vi "ConfigYscales.vi"(4 "Language":refnum<vi>, 5 "曲线自定义封存数组":refnum<vi>, 6 "已选数量":refnum<vi>, 7 "Y轴手配":refnum<vi>, 8 "Y标尺总数":i32, 9 "曲线手配":refnum<vi>, 10 "已选信号列表":refnum<vi>) -> ()   [LabVIEW 2015]
uses:
  Ctrls/btnSeeOrNot.ctl
panel:
  out "txtYlink":string
  out "txtUnit":string
  out "txtCurves":string
  out "txtYVisable":string
  out "txtSignal":string
  out "txtRename":string
  out "txtYName":string
  out "txtYsn":string
  out "txtYSetupTitle":string caption="txtYSetup"
  out "txtCurvesSetup":string
  in  "btnSaveCurvesSetup":bool
  in  "曲线配置簇数组":T1(array[cluster]) {"关联Y轴" min=1 max=8 format="Y轴%d"; "曲线序号" format="曲线%d"}
  in  "btnSaveYsetup":bool
  in  "btnExit":bool
  in  "曲线簇":T2={"曲线序号"=0, "SignalName"="", "SignalTag"="", "自定义名"="", "单位"="", "关联Y轴"=1} {"关联Y轴" min=1 max=8 format="Y轴%d"; "曲线序号" format="曲线%d"}
  in  "Y簇":cluster{"Y轴名称 2":string, "Y轴序号 2":i32, "可见性":T3} {"Y轴序号 2" format="Y轴%d"}
  in  "Y轴配置":T4(array[cluster]) {"Y轴序号 2" format="Y轴%d"}
  in  "曲线配置簇":T2
  in  "Y轴配置簇":cluster{"Y轴序号":u8, "Y轴名称":string, "可见性":bool}
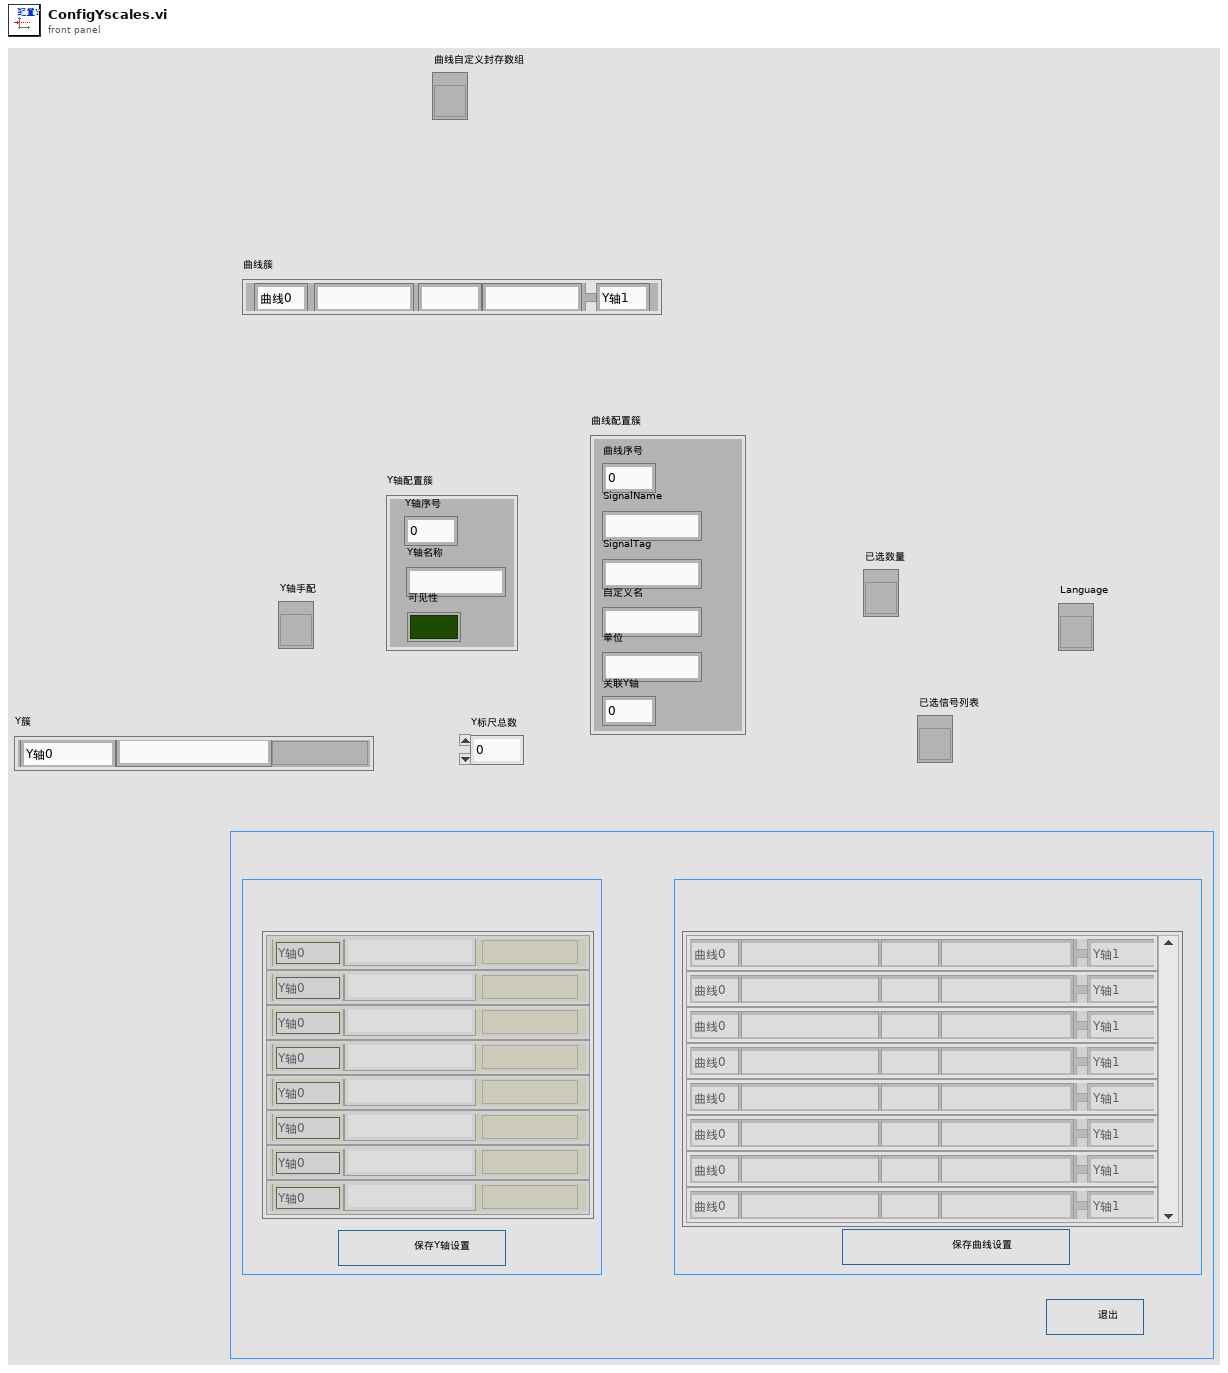
[diagram p1: front panel]
types:
  T1 = cluster{"曲线序号":u8, "SignalName":string, "SignalTag":string, "自定义名":string, "单位":string, "关联Y轴":u8}[]
  T2 = cluster{"曲线序号":u8, "SignalName":string, "SignalTag":string, "自定义名":string, "单位":string, "关联Y轴":u8}
  T3 = typedef "btnSeeOrNot.ctl" = bool
  T4 = cluster{"Y轴名称 2":string, "Y轴序号 2":i32, "可见性":T3}[]
  T5 = enum8{"Enabled", "Disabled", "Disabled and Grayed Out"}
  T6 = typedef "可不可见.ctl" = bool
  T7 = cluster{"Y轴名称 2":string, "Y轴序号 2":i32, "可见性":T6}[]
  T8 = cluster{"曲线序号":u8, "SignalName":string, "SignalTag":string, "自定义名":string, "单位":string, "关联Y轴":u8, "插值方式":dbl}[]
  T9 = cluster{"曲线序号":u8, "SignalName":string, "SignalTag":string, "自定义名":string, "单位":string, "关联Y轴":u8, "插值方式":dbl}
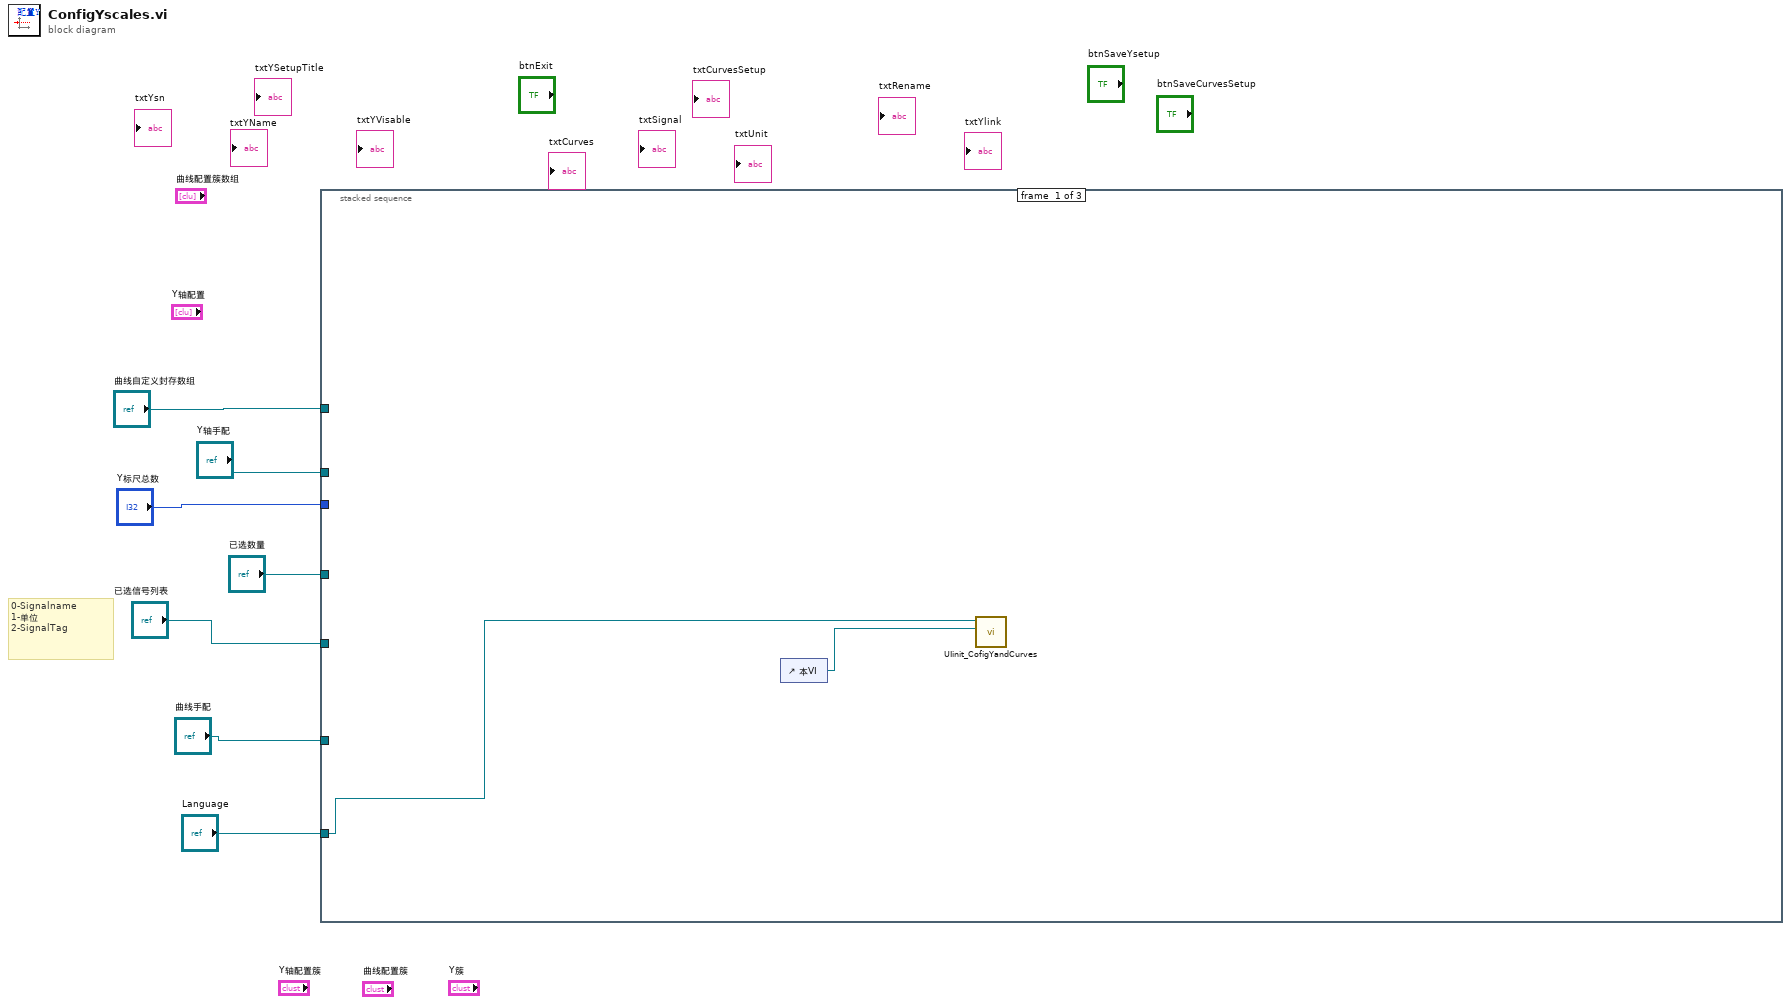
[diagram p0: block diagram]
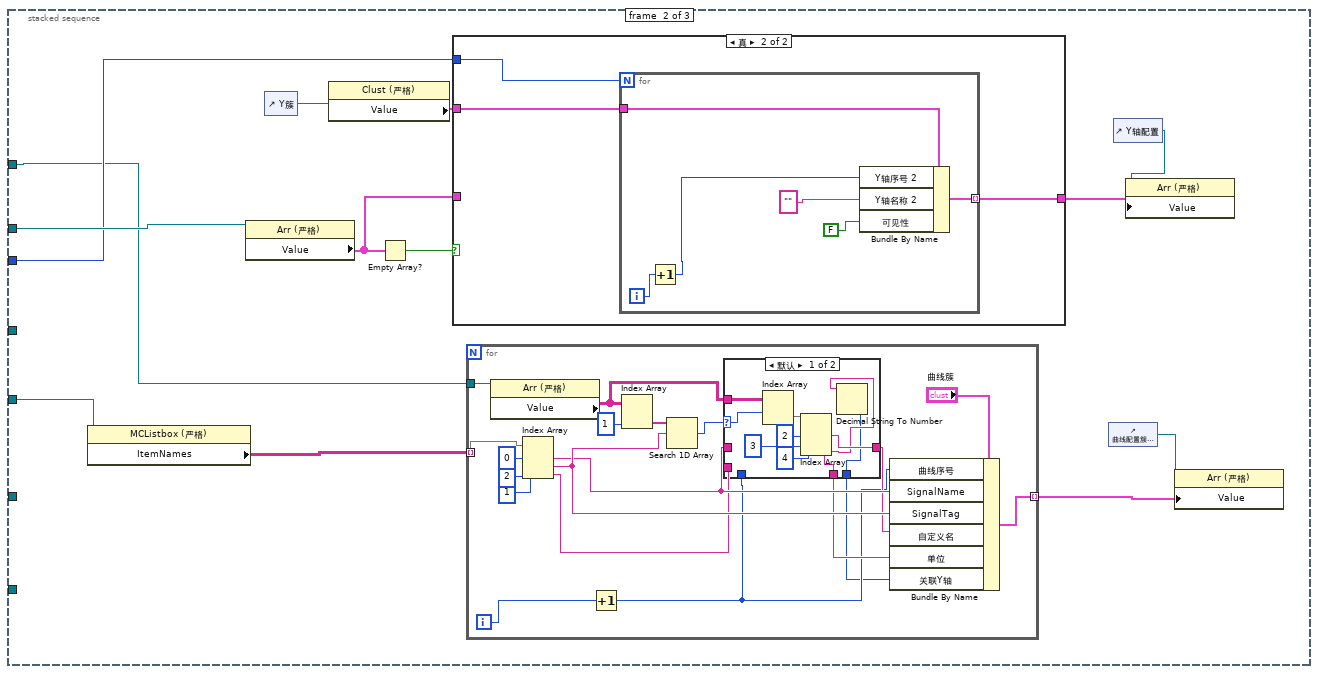
[diagram p2: hidden frame]
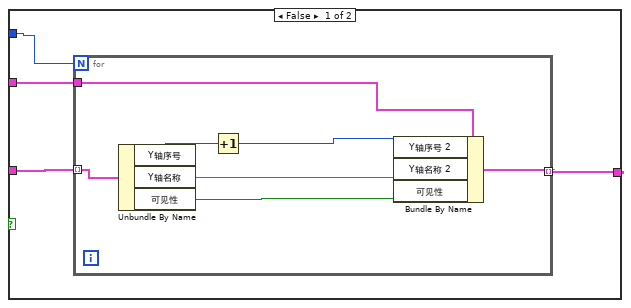
[diagram p4: hidden frame]
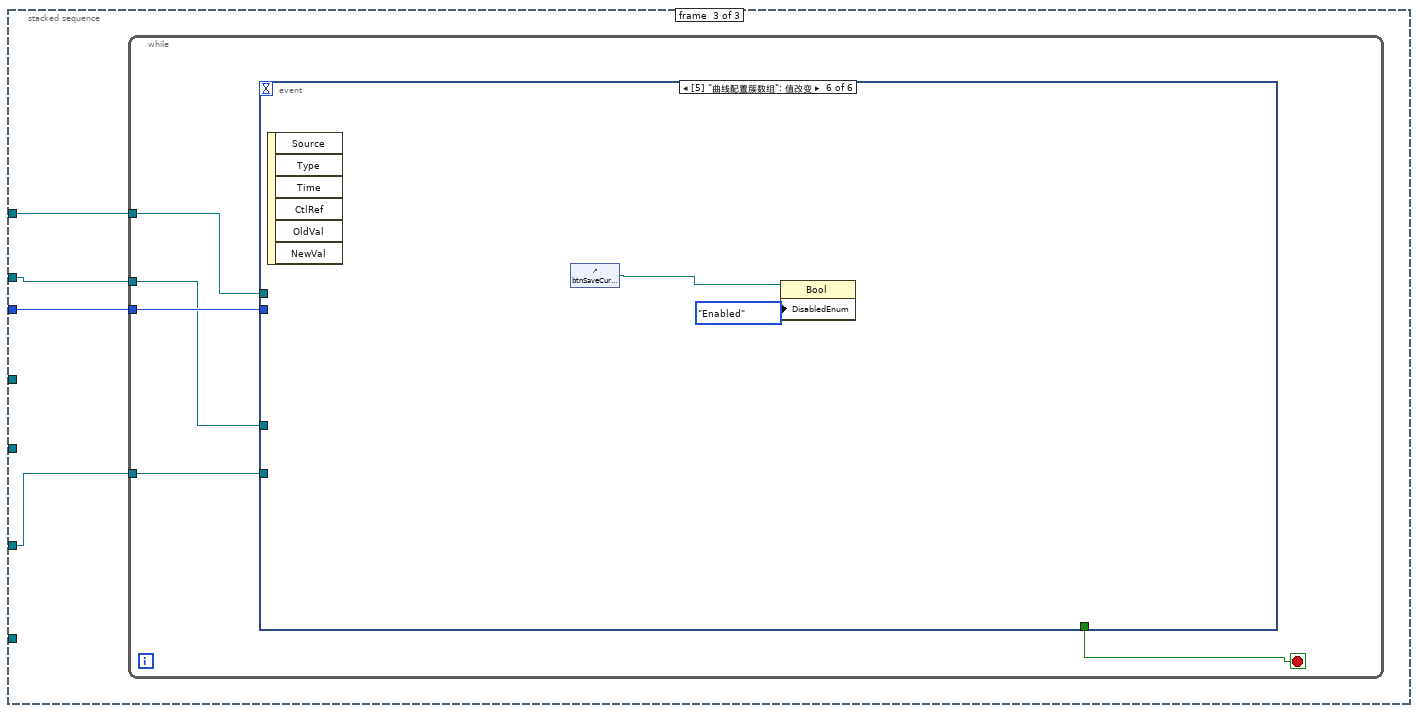
[diagram p5: hidden frame]
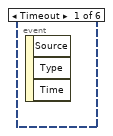
[diagram p6: hidden frame]
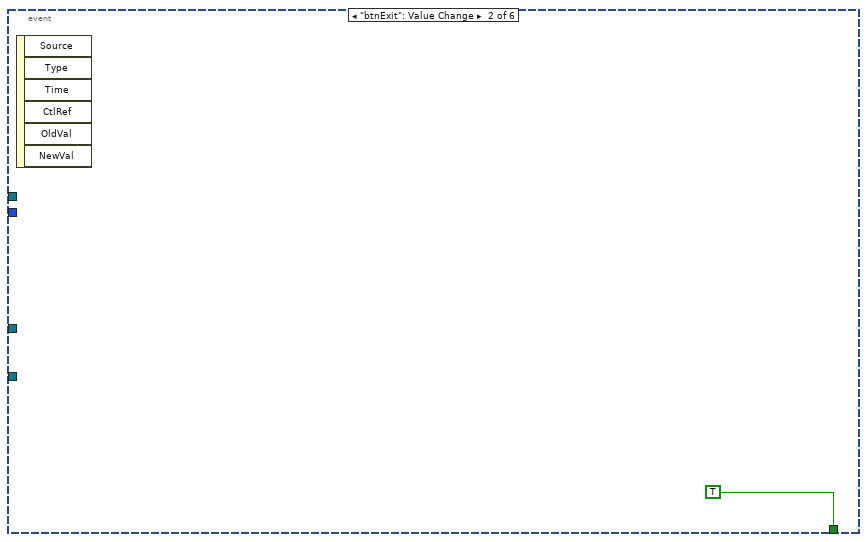
[diagram p7: hidden frame]
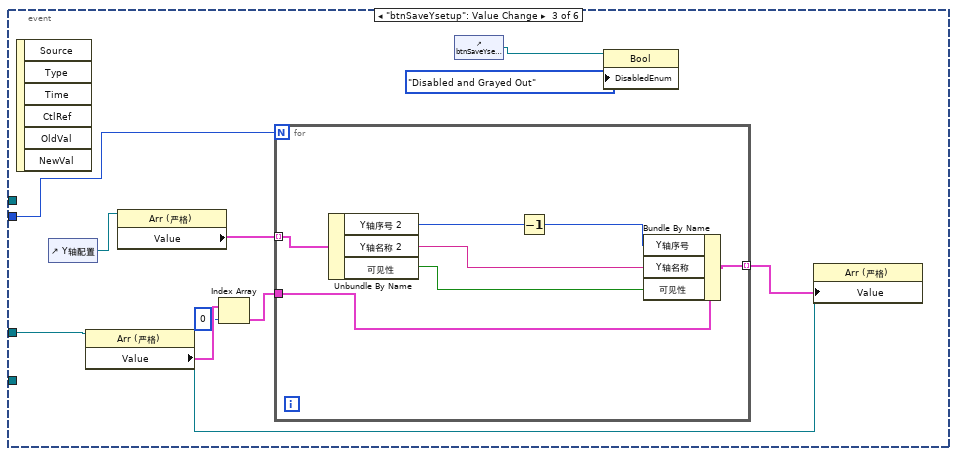
[diagram p8: hidden frame]
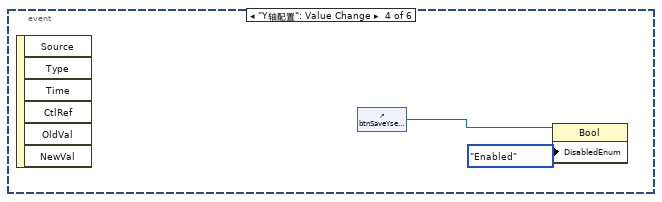
[diagram p9: hidden frame]
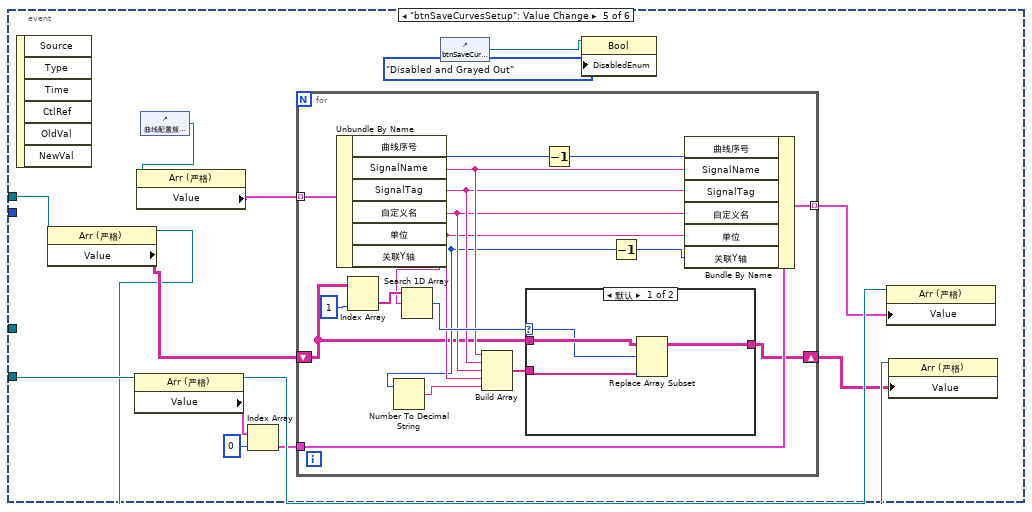
[diagram p10: hidden frame]
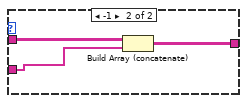
[diagram p11: hidden frame]
diagram:
  # "0-Signalname\n1-单位\n2-SignalTag"
  n1 = stacked-sequence {
    tunnel: "Y标尺总数" -> [_ w15 w77]
    tunnel: "已选信号列表" -> [_ w12 _]
    tunnel: "Y轴手配" -> [_ w22 w76]
    tunnel: "曲线自定义封存数组" -> [_ w10 w78]
    tunnel: "曲线手配" -> [_ _ w75]
    tunnel: "已选数量" -> [_ _ _]
    tunnel: "Language" -> [w9 _ _]
    frame #0 {
      n2 = control-ref of="本VI"() -> (w8:refnum<vi>)
      n3 = call "UIinit_CofigYandCurves.vi"("VIref"=w8, "Language"=w9) -> ()  [unwired: 10 in]
    }
    frame #1 {
      n4 = property class="MCListbox (严格)"(reference=w12) -> ("ItemNames"=w11:string[][])  [unwired: 1 in, 2 out]
      n5 = property class="Arr (严格)"(reference=w22) -> ("Value"=w20:cluster{"Y轴序号":u8, "Y轴名称":string, "可见性":bool}[])  [unwired: 1 in, 2 out]
      n6 = control-ref of="Y簇"() -> (w17:refnum<vi>)
      n7 = property class="Clust (严格)"(reference=w17) -> ("Value"=w16:cluster{"Y轴名称 2":string, "Y轴序号 2":i32, "可见性":T6})  [unwired: 1 in, 2 out]
      n8 = Empty Array?(array=w20) -> (empty?=w21:bool)
      n9 = case shown="真" w21 {
        tunnel: w20 -> [w58 _]
        tunnel: [w57 w66] -> w18
        tunnel: w16 -> [w56 w67]
        tunnel: w15 -> [w55 w68]
        frame False {
          n10 = for {
            N: w55 -> [_]
            tunnel: w58 -> [w65] mode=indexing
            tunnel: [w61] -> w57 mode=indexing
            tunnel: w56 -> [w60]
            n11 = Unbundle By Name(w65) -> ("Y轴序号"=w64:u8, "Y轴名称"=w62:string, "可见性"=w63:bool)
            n12 = Increment(x=w64) -> (x+1=w59:u8)
            n13 = Bundle By Name(cluster=w60, "Y轴序号 2"=w59, "Y轴名称 2"=w62, "可见性"=w63) -> (w61:cluster{"Y轴名称 2":string, "Y轴序号 2":i32, "可见性":T6})
          }
        }
        frame True {
          n14 = for {
            N: w68 -> [_]
            tunnel: w67 -> [w74]
            tunnel: [w73] -> w66 mode=indexing
            i -> [w72]
            n15 = Increment(x=w72) -> (x+1=w69:i32)
            n16 = Bundle By Name(cluster=w74, "Y轴序号 2"=w69, "Y轴名称 2"="", "可见性"=FALSE) -> (w73:cluster{"Y轴名称 2":string, "Y轴序号 2":i32, "可见性":T6})
          }
        }
      }
      n17 = for {
        tunnel: [w39] -> w13 mode=indexing
        tunnel: w11 -> [w38] mode=indexing
        tunnel: w10 -> [w34]
        i -> [w40]
        n18 = property class="Arr (严格)"(reference=w34) -> ("Value"=w25:string[][])  [unwired: 1 in, 2 out]
        n19 = Index Array(array=w38, index #1=0 ("索引"), index #2=2 ("索引"), index #3=1 ("索引")) -> (element #1=w29:string, element #2=w31:string, element #3=w27:string)
        n20 = Increment(x=w40) -> (x+1=w24:i32)
        n21 = Index Array(array=w25, index (col)=1 ("禁用的索引 (列)")) -> (element=w32:string[])  [unwired: 1 in]
        n22 = Search 1D Array(1D array=w32, element=w31) -> (index of element=w30:i32)  [unwired: 1 in]
        n23 = case shown="默认" w30 {
          selector: w30 -> [w50 _]
          tunnel: w29 -> [_ w54]
          tunnel: [w46 w54] -> w28
          tunnel: w27 -> [_ w53]
          tunnel: [w45 w53] -> w26
          tunnel: w25 -> [w51 _]
          tunnel: w24 -> [_ w52]
          tunnel: [w42 w52] -> w23
          frame Default {
            n24 = Index Array(array=w51, index (row)=w50) -> (element=w49:string[])  [unwired: 1 in]
            n25 = Index Array(array=w49, index #1=2 ("索引"), index #2=3 ("索引"), index #3=4 ("索引")) -> (element #1=w46:string, element #2=w45:string, element #3=w43:string)
            n26 = Decimal String To Number(string=w43) -> (number=w42:i32)  [unwired: 2 in, 1 out]
          }
          frame -1 {
          }
        }
        n27 = Bundle By Name(cluster="曲线簇", "曲线序号"=w24, "SignalName"=w29, "SignalTag"=w31, "自定义名"=w28, "单位"=w26, "关联Y轴"=w23) -> (w39:T2)
      }
      n28 = control-ref of="曲线配置簇数组"() -> (w14:refnum<vi>)
      n29 = control-ref of="Y轴配置"() -> (w19:refnum<vi>)
      n30 = property class="Arr (严格)"(reference=w19, "Value"=w18) -> ()  [unwired: 1 in, 2 out]
      n31 = property class="Arr (严格)"(reference=w14, "Value"=w13) -> ()  [unwired: 1 in, 2 out]
    }
    frame #2 {
      n32 = while {
        tunnel: w78 -> [w82]
        tunnel: w77 -> [w81]
        tunnel: w76 -> [w80]
        tunnel: w75 -> [w79]
        stop <- w83 stop-if-true
        n33 = event shown="[5] \"曲线配置簇数组\": 值改变" {
          selector: _ -> [_ _ _ _ _ _]
          dyn-events: _ -> [_ _ _ _ _ _]
          timeout: _ -> [_ _ _ _ _ _]
          tunnel: [_ TRUE _ _ _ _] -> w83
          tunnel: w82 -> [_ _ _ _ w110 _]
          tunnel: w81 -> [_ _ w93 _ _ _]
          tunnel: w80 -> [_ _ w92 _ _ _]
          tunnel: w79 -> [_ _ _ _ w114 _]
          event Timeout {
            n34 = event-data() -> ()  [unwired: 1 in, 3 out]
          }
          event "btnExit": Value Change {
            n35 = event-data() -> ()  [unwired: 1 in, 6 out]
          }
          event "btnSaveYsetup": Value Change {
            n36 = event-data() -> ()  [unwired: 1 in, 6 out]
            n37 = control-ref of="Y轴配置"() -> (w95:refnum<vi>)
            n38 = property class="Arr (严格)"(reference=w92) -> (reference out=w88:refnum<vi>, "Value"=w91:cluster{"Y轴序号":u8, "Y轴名称":string, "可见性":bool}[])  [unwired: 1 in, 1 out]
            n39 = property class="Arr (严格)"(reference=w95) -> ("Value"=w94:T7)  [unwired: 1 in, 2 out]
            n40 = Index Array(array=w91, index=0 ("索引")) -> (element=w89:cluster{"Y轴序号":u8, "Y轴名称":string, "可见性":bool})
            n41 = for {
              N: w93 -> [_]
              tunnel: w94 -> [w102] mode=indexing
              tunnel: w89 -> [w101]
              tunnel: [w97] -> w87 mode=indexing
              n42 = Unbundle By Name(w102) -> ("Y轴序号 2"=w96:i32, "Y轴名称 2"=w99:string, "可见性"=w98:T6)
              n43 = Decrement(x=w96) -> (x-1=w100:i32)
              n44 = Bundle By Name(cluster=w101, "Y轴序号"=w100, "Y轴名称"=w99, "可见性"=w98) -> (w97:cluster{"Y轴序号":u8, "Y轴名称":string, "可见性":bool})
            }
            n45 = control-ref of="btnSaveYsetup"() -> (w85:refnum<vi>)
            n46 = property class="Bool"(reference=w85, "DisabledEnum"=T5."Disabled and Grayed Out" ("禁用")) -> ()  [unwired: 1 in, 2 out]
            n47 = property class="Arr (严格)"(reference=w88, "Value"=w87) -> ()  [unwired: 1 in, 2 out]
          }
          event "Y轴配置": Value Change {
            n48 = event-data() -> ()  [unwired: 1 in, 6 out]
            n49 = control-ref of="btnSaveYsetup"() -> (w103:refnum<vi>)
            n50 = property class="Bool"(reference=w103, "DisabledEnum"=T5."Enabled" ("禁用")) -> ()  [unwired: 1 in, 2 out]
          }
          event "btnSaveCurvesSetup": Value Change {
            n51 = event-data() -> ()  [unwired: 1 in, 6 out]
            n52 = property class="Arr (严格)"(reference=w110) -> (reference out=w108:refnum<vi>, "Value"=w109:string[][])  [unwired: 1 in, 1 out]
            n53 = property class="Arr (严格)"(reference=w114) -> (reference out=w113:refnum<vi>, "Value"=w115:T8)  [unwired: 1 in, 1 out]
            n54 = control-ref of="曲线配置簇数组"() -> (w118:refnum<vi>)
            n55 = property class="Arr (严格)"(reference=w118) -> ("Value"=w117:T1)  [unwired: 1 in, 2 out]
            n56 = Index Array(array=w115, index=0 ("索引")) -> (element=w111:T9)
            n57 = for {
              tunnel: w117 -> [w136] mode=indexing
              tunnel: [w134] -> w112 mode=indexing
              tunnel: w111 -> [w133]
              shift-right: [w121] -> w107
              shift-left: w109 -> [w122]
              n58 = Unbundle By Name(w136) -> ("曲线序号"=w120:u8, "SignalName"=w129:string, "SignalTag"=w128:string, "自定义名"=w127:string, "单位"=w126:string, "关联Y轴"=w124:u8)
              n59 = Index Array(array=w122, index (col)=1 ("禁用的索引 (列)")) -> (element=w130:string[])  [unwired: 1 in]
              n60 = Number To Decimal String(number=w124) -> (decimal integer string=w125:string)  [unwired: 1 in]
              n61 = Search 1D Array(1D array=w130, element=w128) -> (index of element=w132:i32)  [unwired: 1 in]
              n62 = Build Array(w129, w128, w127, w126, w125) -> (w123:string[])
              n63 = case shown="默认" w132 {
                selector: w132 -> [w138 _]
                tunnel: w123 -> [w139 w142]
                tunnel: w122 -> [w140 w143]
                tunnel: [w137 w141] -> w121
                frame Default {
                  n64 = Replace Array Subset(array=w140, new element=w139, index (row)=w138) -> (w137:string[][])  [unwired: 1 in]
                }
                frame -1 {
                  n65 = Build Array (concatenate)(w143, w142) -> (w141:string[][])
                }
              }
              n66 = Decrement(x=w120) -> (x-1=w119:u8)
              n67 = Decrement(x=w124) -> (x-1=w135:u8)
              n68 = Bundle By Name(cluster=w133, "曲线序号"=w119, "SignalName"=w129, "SignalTag"=w128, "自定义名"=w127, "单位"=w126, "关联Y轴"=w135) -> (w134:T9)
            }
            n69 = control-ref of="btnSaveCurvesSetup"() -> (w106:refnum<vi>)
            n70 = property class="Bool"(reference=w106, "DisabledEnum"=T5."Disabled and Grayed Out" ("禁用")) -> ()  [unwired: 1 in, 2 out]
            n71 = property class="Arr (严格)"(reference=w113, "Value"=w112) -> ()  [unwired: 1 in, 2 out]
            n72 = property class="Arr (严格)"(reference=w108, "Value"=w107) -> ()  [unwired: 1 in, 2 out]
          }
          event "曲线配置簇数组": Value Change {
            n73 = event-data() -> ()  [unwired: 1 in, 6 out]
            n74 = control-ref of="btnSaveCurvesSetup"() -> (w144:refnum<vi>)
            n75 = property class="Bool"(reference=w144, "DisabledEnum"=T5."Enabled" ("禁用")) -> ()  [unwired: 1 in, 2 out]
          }
        }
      }
    }
  }
